vi "STAT_OPER.vi"(8 "error in":errorcluster) -> (0 "error out":errorcluster, 3 "f_all_data":dbl[](array[numeric]))   [LabVIEW 2023]
panel:
  out "data out":string
  out "All_data":i32[](array[numeric])
  in  "TCPIPin":T1={"address"="192.168.100.111", "remote port or service name"=5025, "timeout ms (60000)"=10000}
  # "CLC_Gen4_L2"
  # "AiP_1 : 0\nAiP_2 : 1\nAiP_3 : 2\nAiP_4 : 3\nAiP_5 : 4\nAiP_6 : 5\nAiP_7 : 6\nAiP_8 : 7"
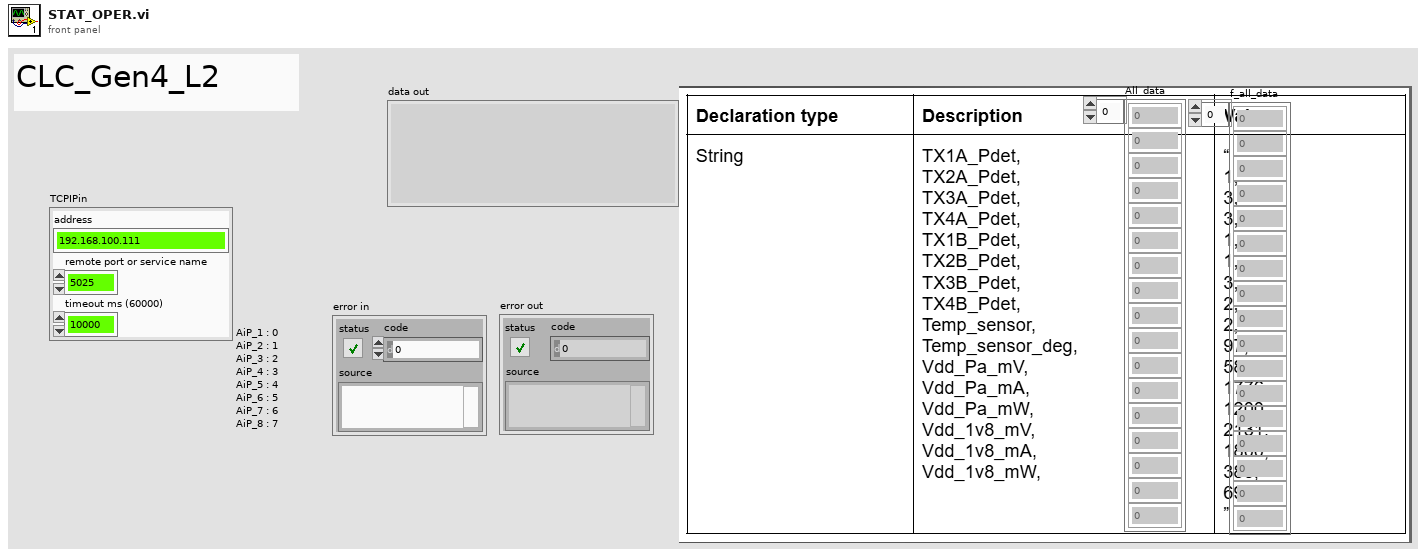
[diagram p1: front panel]
types:
  T1 = cluster{"address":string, "remote port or service name":u16, "timeout ms (60000)":i32}
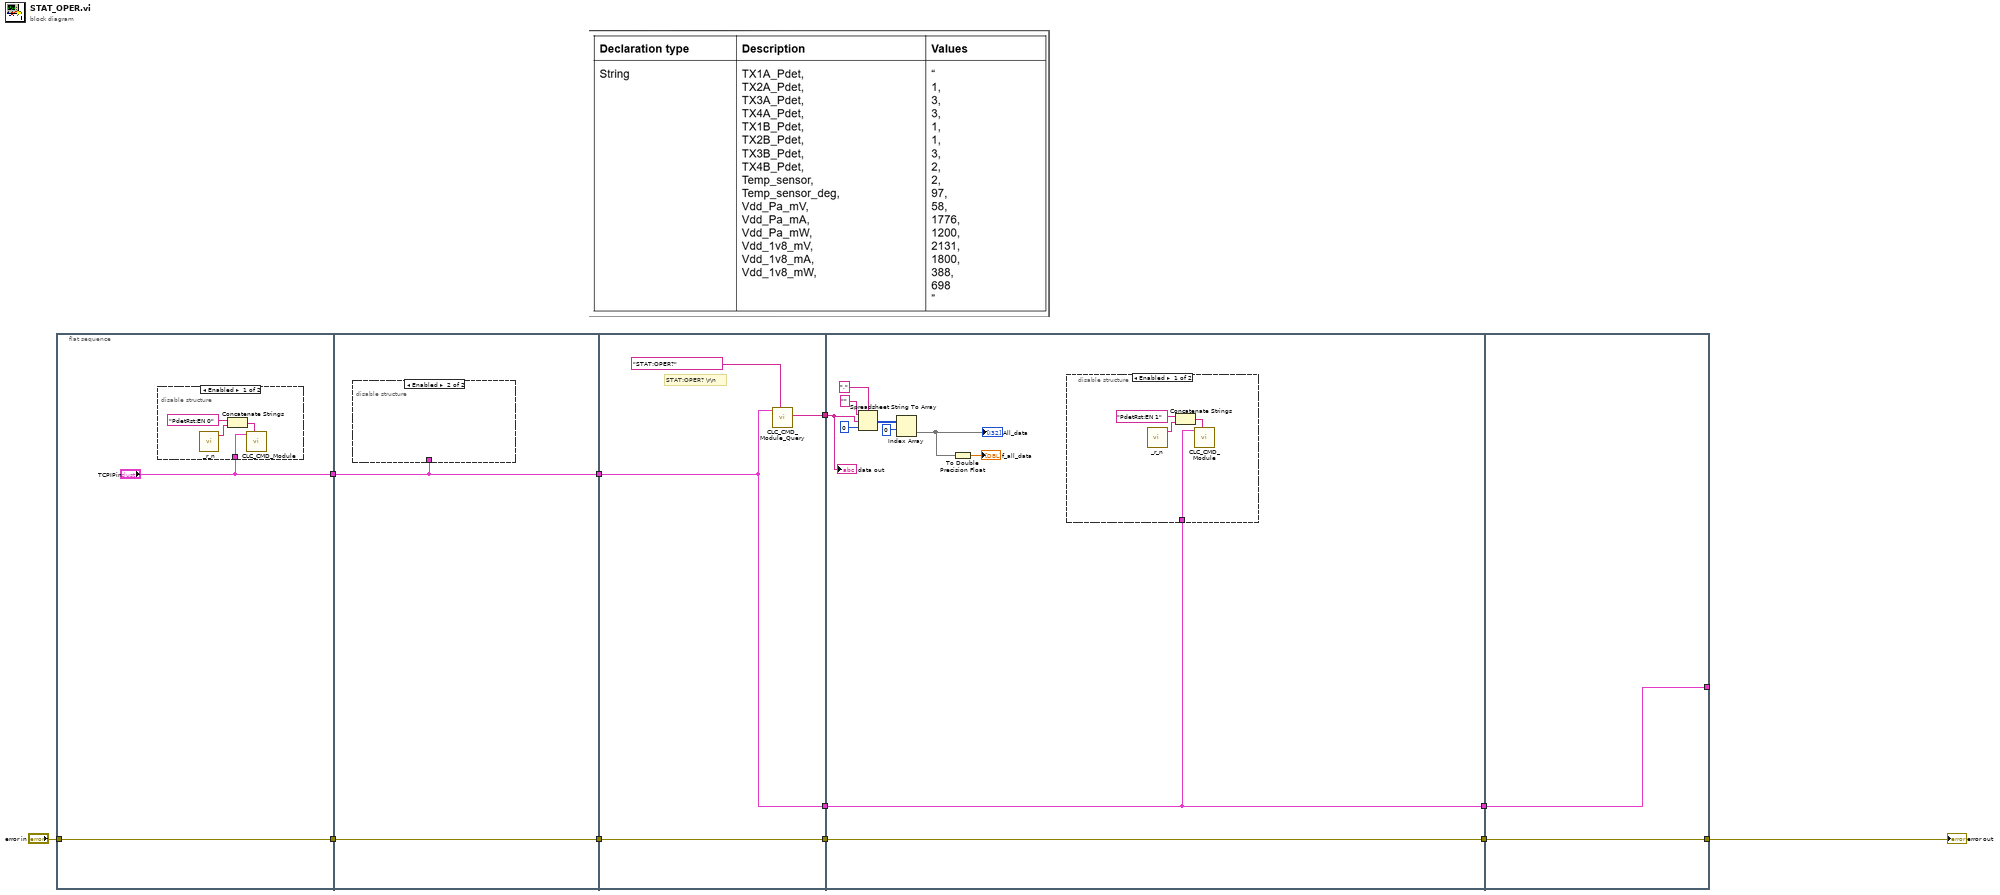
[diagram p0: block diagram]
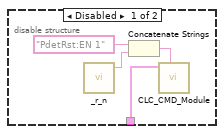
[diagram p3: hidden frame]
diagram:
  n1 = flat-sequence {
    tunnel: ["TCPIPin"] -> w4
    tunnel: "error in" -> [w13]
    tunnel: [w13] -> w2
    tunnel: w4 -> [w18]
    tunnel: [w18] -> w3
    tunnel: w2 -> [w19]
    tunnel: [w19] -> w1
    tunnel: [w27] -> w11
    tunnel: [w26] -> w10
    tunnel: w3 -> [w26]
    tunnel: [w25] -> w6
    tunnel: w1 -> [w25]
    tunnel: w11 -> [w35]
    tunnel: w10 -> [w30]
    tunnel: [w30] -> w9
    tunnel: [w31] -> w7
    tunnel: w6 -> [w31]
    tunnel: [w43] -> _
    tunnel: w9 -> [w43]
    tunnel: [w42] -> w5
    tunnel: w7 -> [w42]
    frame #0 {
      n2 = disable-structure shown="Enabled" {
        disable-tunnel: "TCPIPin" -> [w14 _]
        frame Enabled {
          n3 = call "_r_n.vi"() -> ("command"=w16:string)  [unwired: 5 in]
          n4 = Concatenate Strings("PdetRst:EN 0" ("CMD in"), w16) -> (w15:string)
          n5 = call "CLC_CMD_Module.vi"("CMD in"=w15, "TCPIPin"=w14) -> ()  [unwired: 6 in, 4 out]
        }
        frame Disabled {
        }
      }
    }
    frame #1 {
      n6 = disable-structure shown="Enabled" {
        disable-tunnel: w18 -> [w20 _]
        frame Disabled {
          n7 = call "_r_n.vi"() -> ("command"=w21:string)  [unwired: 5 in]
          n8 = Concatenate Strings("PdetRst:EN 1" ("CMD in"), w21) -> (w22:string)
          n9 = call "CLC_CMD_Module.vi"("CMD in"=w22, "TCPIPin"=w20) -> ()  [unwired: 6 in, 4 out]
        }
        frame Enabled {
        }
      }
    }
    frame #2 {
      # "STAT:OPER? \\r\\n"
      n10 = call "CLC_CMD_Module_Query.vi"("CMD in"="STAT:OPER?" ("data in"), "TCPIPin"=w26) -> ("data out"=w27:string)  [unwired: 7 in, 2 out]
    }
    frame #3 {
      n11 = Spreadsheet String To Array(delimiter (Tab)=",", format string="", spreadsheet string=w35, array type (2D Dbl)=0) -> (array=w32:i32[][])
      n12 = Index Array(array=w32, index (row)=0 ("disabled index (col)")) -> (element=w29:i32[])  [unwired: 1 in]
      "All_data" <- w29
      n13 = To Double Precision Float(number=w29) -> (double precision float=→"f_all_data":dbl[])
      n14 = disable-structure shown="Enabled" {
        disable-tunnel: w30 -> [w38 _]
        frame Enabled {
          n15 = call "_r_n.vi"() -> ("command"=w41:string)  [unwired: 5 in]
          n16 = Concatenate Strings("PdetRst:EN 1" ("CMD in"), w41) -> (w40:string)
          n17 = call "CLC_CMD_Module.vi"("CMD in"=w40, "TCPIPin"=w38) -> ()  [unwired: 6 in, 4 out]
        }
        frame Disabled {
        }
      }
      "data out" <- w35
    }
    frame #4 {
    }
  }
  "error out" <- w5
